vi "当前时间格式显示 (子VI).vi"() -> (3 "当前时间格式显示":string)   [LabVIEW 2016]
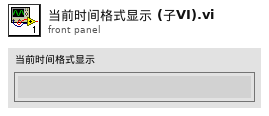
[diagram p1: front panel]
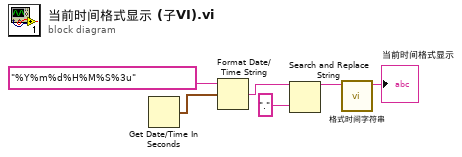
[diagram p0: block diagram]
diagram:
  n1 = Get Date/Time In Seconds() -> (seconds since 1Jan1904=w1:timestamp)
  n2 = Format Date/Time String(time format string (%c)="%Y%m%d%H%M%S%3u" ("时间格式字符串(%c)"), seconds (now)=w1) -> (date/time string=w5:string)  [unwired: 1 in]
  n3 = Search and Replace String(input string=w5, search string="." ("搜索字符串")) -> (result string=w4:string)  [unwired: 6 in, 3 out]
  n4 = call "格式时间字符串.vi"("字符串"=w4) -> ("连接的字符串"=→"当前时间格式显示":string)  [unwired: 10 in]
